vi "Array of Typedef Enum - Should Pass.vi"() -> ()   [LabVIEW 2017, in "Transparent Assertions.Tests.lvlib" / "Assert Collection Contains.lvlib"]
uses:
  Assert Collection Contains.lvlib
  Enum Typedef.ctl
  src/Transparent Assertions/Transparent Assertions.lvlib
panel:
  out "error out":errorcluster
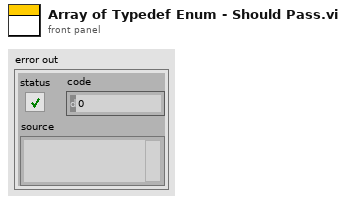
[diagram p1: front panel]
types:
  T1 = typedef "Transparent Assertions.Tests.lvlib/Assert Collection Contains.lvlib/Enum Typedef.ctl" = enum16{"One", "Two", "Three"}
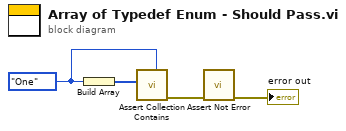
[diagram p0: block diagram]
diagram:
  w3 = Enum_Typedef."One" ("Enum")
  n1 = Build Array(w3) -> (w4:T1[])
  n2 = call "Assert Collection Contains.vi"("Expected"=w3, "Collection"=w4) -> ("error out"=w2:errorcluster)  [unwired: 9 in]
  n3 = call "Assert Not Error.vi"("error in (no error)"=w2) -> ("error out"=→"error out":errorcluster)  [unwired: 10 in]
